vi "AgPSA _Read Trace (loop delay override).vi"(6 "loop delay (ms)":u32=1000, 8 "error in (no error)":errorcluster, 9 "Maximum Time (10000 ms)":i32=10000, 10 "Trace Name (1: Trace 1)":u16(ring)=1 items=["Trace 1"=1, "Trace 2"=2, "Trace 3"=3], 11 "VISA resource name":refnum<visa-resource-name>) -> (0 "error out":errorcluster, 2 "Trace Waveform":T1(graph), 3 "VISA resource name out":refnum<visa-resource-name>)   [LabVIEW 2015]
uses:
  <instrlib>/Agilent ESA PSA Series/Agilent ESA PSA Series.lvlib
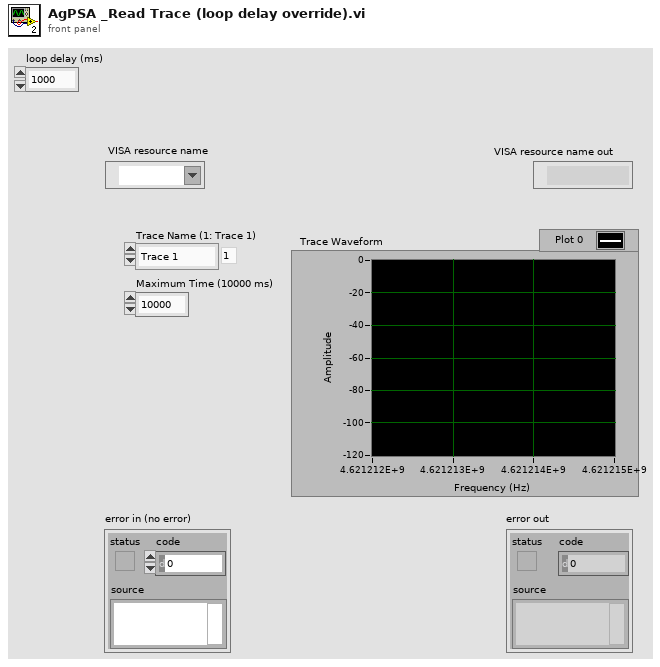
[diagram p1: front panel]
types:
  T1 = cluster{"Initial X":dbl, "X Increment":dbl, "Trace Array":dbl[]}
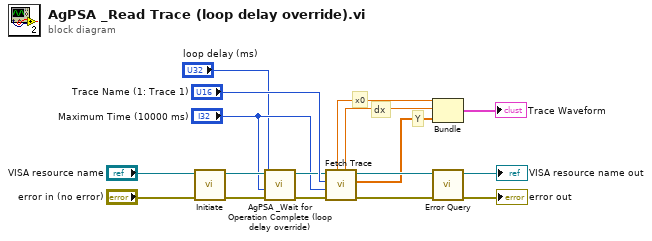
[diagram p0: block diagram]
diagram:
  # "Y"
  # "dx"
  # "x0"
  n1 = call <instrlib>:"Initiate.vi"("error in (no error)"="error in (no error)", "VISA resource name"="VISA resource name") -> ("error out"=w5:errorcluster, "VISA resource name out"=w6:refnum<visa-resource-name>)  [unwired: 8 in]
  n2 = call "AgPSA _Wait for Operation Complete (loop delay override).vi"("error in (no error)"=w5, "Maximum Time (10000ms)"="Maximum Time (10000 ms)", "loop delay (ms)"="loop delay (ms)", "VISA resource name"=w6) -> ("error out"=w3:errorcluster, "VISA resource name out"=w4:refnum<visa-resource-name>)  [unwired: 6 in]
  n3 = call <instrlib>:"Fetch Trace.vi"("error in (no error)"=w3, "Timeout (10000 ms)"="Maximum Time (10000 ms)", "Trace Name (1: Trace 1)"="Trace Name (1: Trace 1)", "VISA resource name"=w4) -> ("error out"=w15:errorcluster, "Trace Array"=w10:dbl[], "VISA resource name out"=w17:refnum<visa-resource-name>, "X Increment"=w13:dbl, "Initial X"=w12:dbl)  [unwired: 3 in]
  n4 = Bundle("Initial X"=w12, "X Increment"=w13, "Trace Array"=w10) -> (→"Trace Waveform":T1)  [unwired: 1 in]
  n5 = call <instrlib>:"Error Query.vi"("error in (no error)"=w15, "VISA resource name"=w17) -> ("error out"=→"error out":errorcluster, "VISA resource name out"=→"VISA resource name out":refnum<visa-resource-name>)  [unwired: 6 in, 2 out]
